vi "ServerUDP.vi"() -> ()   [LabVIEW 2025]
panel:
  out "seconds since 1Jan1904":timestamp
  out "Waveform Graph":dbl[](graph)
  out "finish":bool
  out "output cluster":T1
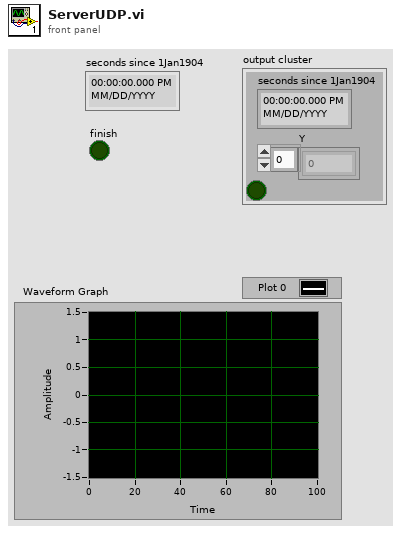
[diagram p1: front panel]
types:
  T1 = typedef "Wiasomoœæ_c.ctl" = cluster{"seconds since 1Jan1904":timestamp, "Y":dbl[], bool}
  T2 = cluster{"seconds since 1Jan1904":timestamp, "Y":dbl[], bool}
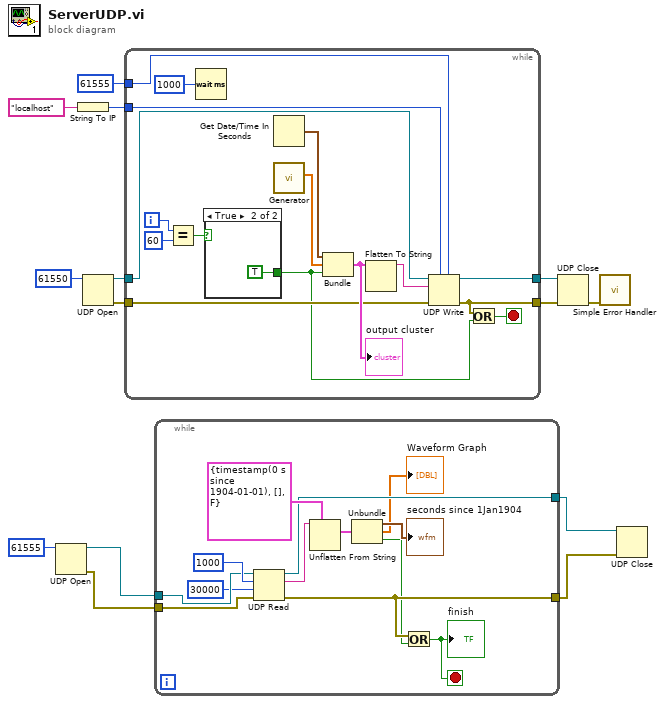
[diagram p0: block diagram]
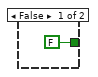
[diagram p2: hidden frame]
diagram:
  n1 = UDP Open(11:u16 61555 ("port")) -> (port=w4:refnum<k16>, 0:w2:errorcluster)  [unwired: 4 in, 1 out]
  n2 = String To IP(1:"localhost" ("name")) -> (0:w11:u32)
  n3 = UDP Open(11:u16 61550 ("port")) -> (port=w14:refnum<k16>, 0:w8:errorcluster)  [unwired: 4 in, 1 out]
  n4 = while {
    tunnel: w14 -> [w26]
    tunnel: [w25] -> w13
    tunnel: w11 -> [w23]
    tunnel: 61555 -> [w22]
    tunnel: w8 -> [w21]
    tunnel: [w20] -> w7
    i -> [w19]
    stop <- w24 stop-if-true
    n5 = Equal?(x=w19, y=60) -> (x = y?=w17:bool)
    n6 = Wait (ms)(milliseconds to wait=u32 1000) -> ()  [unwired: 1 out]
    n7 = case shown="True" w17 {
      tunnel: [FALSE TRUE] -> w16
      frame False {
      }
      frame True {
      }
    }
    n8 = Get Date/Time In Seconds() -> (seconds since 1Jan1904=w30:timestamp)
    n9 = call "Generator.vi"() -> ("Y"=w29:dbl[])  [unwired: 11 in]
    n10 = Bundle("seconds since 1Jan1904"=w30, "Y"=w29, w16) -> (w28:T2)  [unwired: 1 in]
    "output cluster" <- w28
    n11 = Flatten To String(anything=w28) -> (data string=w27:string)  [unwired: 3 in, 2 out]
    n12 = UDP Write(address=w23, port or service name=w22, connection ID=w26, data in=w27, 8:w21) -> (error out=w20:errorcluster, 3:w25:refnum<k16>)  [unwired: 1 in]
    n13 = Or(x=w20, y=w16) -> (x .or. y?=w24:bool)
  }
  n14 = while {
    tunnel: w4 -> [w42]
    tunnel: [w41] -> w3
    tunnel: w2 -> [w40]
    tunnel: [w39] -> w1
    stop <- w38 stop-if-true
    n15 = UDP Read(connection ID=w42, max size (548)=1000, timeout ms (25000)=30000, 8:w40) -> (data out=w43:string, error out=w39:errorcluster, 3:w41:refnum<k16>)  [unwired: 2 out]
    n16 = Unflatten From String(type=T1 {"seconds since 1Jan1904"=timestamp(0 s since 1904-01-01), "Y"=[], FALSE} ("output cluster"), binary string=w43) -> (value=w37:T1)  [unwired: 3 in, 2 out]
    n17 = Unbundle(w37) -> ("seconds since 1Jan1904"=→"seconds since 1Jan1904":timestamp, "Y"=→"Waveform Graph":dbl[], w34:bool)
    n18 = Or(x=w39, y=w34) -> (x .or. y?=w38:bool)
    "finish" <- w38
  }
  n19 = UDP Close(connection ID=w13, 8:w7) -> (error out=w6:errorcluster)  [unwired: 1 out]
  n20 = call <vilib>:"Simple Error Handler.vi"("error in (no error)"=w6) -> ()  [unwired: 4 in, 5 out]
  n21 = UDP Close(connection ID=w3, 8:w1) -> ()  [unwired: 2 out]
